vi "ReadSZL.vi"() -> ()   [LabVIEW 2020]
uses:
  lib/Snap7.lvlib
panel:
  out "?":string
  out "SZL List":string
  out "Size":i32
  out "ASCII Data":string
  out "Hex Data":string
  out "Running":bool
  out "Status":string="No Error"
  in  "Index":i32 format="%x"
  in  "ID":i32=17 format="%x"
  in  "?":bool
  in  "Slot":i32=2
  in  "Rack":i32
  in  "Address IP":string="192.168.1.12"
  # "SZL Read"
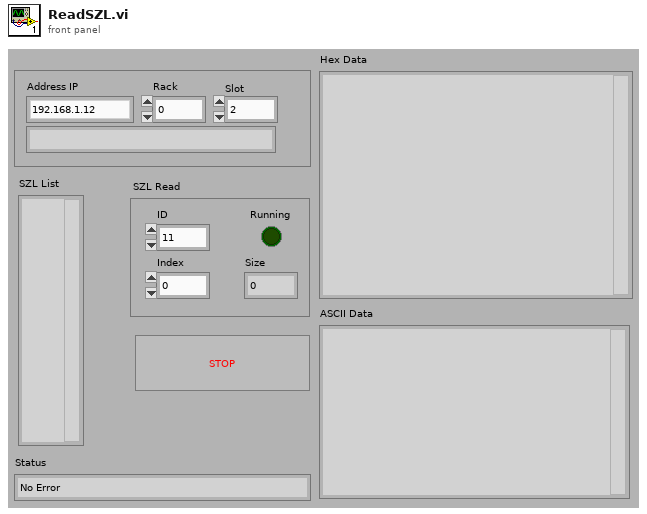
[diagram p1: front panel]
types:
  T1 = enum16{"big-endian, network order", "native, host order", "little-endian"}
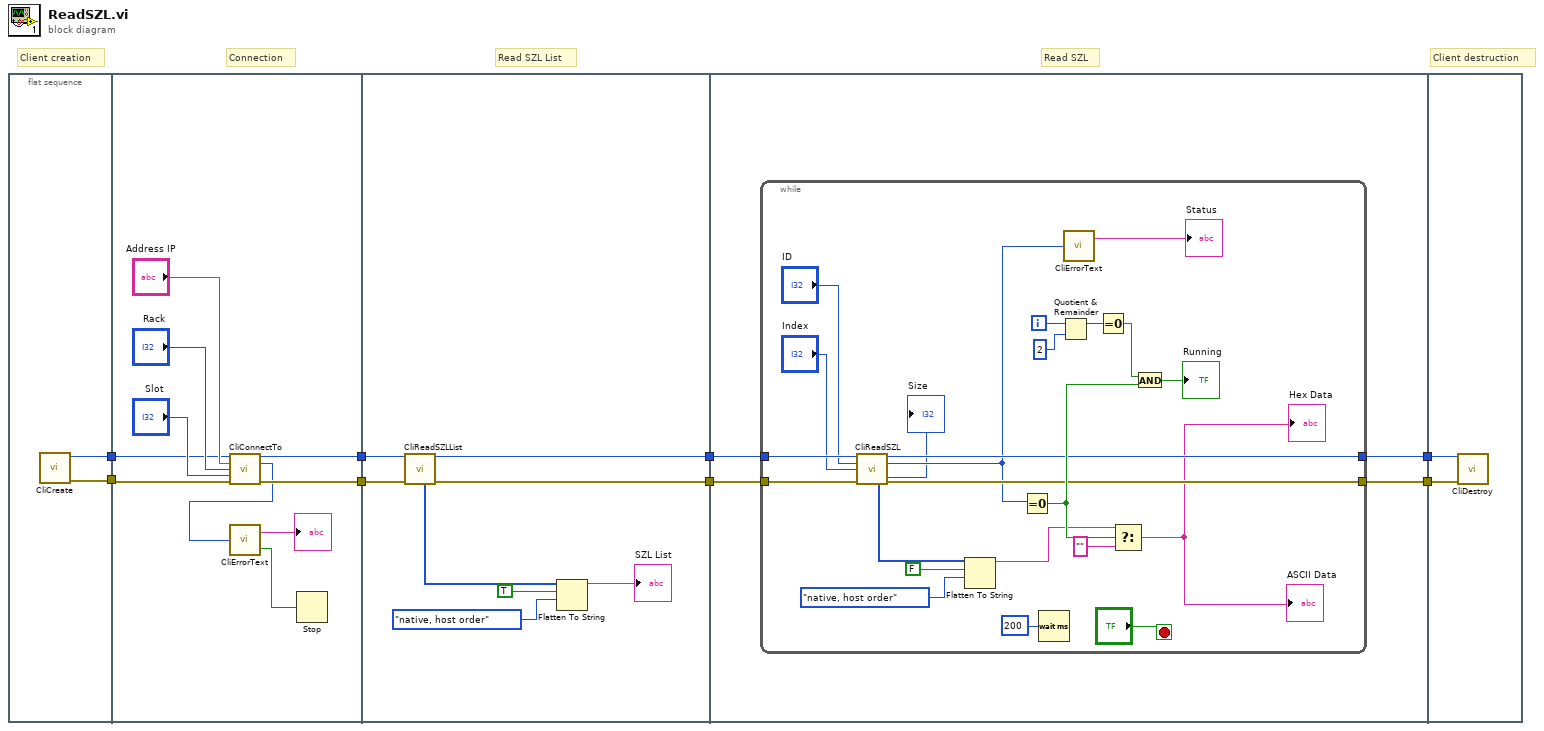
[diagram p0: block diagram]
diagram:
  # "Read SZL List"
  # "Client destruction"
  # "Read SZL"
  # "Connection"
  # "Client creation"
  n1 = flat-sequence {
    tunnel: [w10] -> w8
    tunnel: [w9] -> w7
    tunnel: [w20] -> w4
    tunnel: [w14] -> w2
    tunnel: w8 -> [w16]
    tunnel: w7 -> [w15]
    tunnel: w4 -> [w26]
    tunnel: [w25] -> w3
    tunnel: w2 -> [w28]
    tunnel: [w27] -> w1
    tunnel: w3 -> [w32]
    tunnel: w1 -> [w31]
    tunnel: [w30] -> w6
    tunnel: [w29] -> w5
    tunnel: w6 -> [w57]
    tunnel: w5 -> [w56]
    frame #0 {
      n2 = call "CliCreate.vi"() -> ("ref out"=w10:u64, "error out"=w9:errorcluster)  [unwired: 14 in]
    }
    frame #1 {
      n3 = call "CliConnectTo.vi"("ref in"=w16, "Address"="Address IP", "Rack"="Rack", "Slot"="Slot", "error in (no error)"=w15) -> ("ref out"=w14:u64, "Result"=w12:i32, "error out"=w20:errorcluster)  [unwired: 8 in]
      n4 = call "CliErrorText.vi"("ErrNo"=w12) -> ("Error"=w11:bool, "ErrMessage"=→"?":string)
      n5 = Stop(stop? (T)=w11) -> ()
    }
    frame #2 {
      n6 = call "CliReadSZLList.vi"("ref in"=w28, "error in (no error)"=w26) -> ("ref out"=w27:u64, "List"=w22:u16[], "error out"=w25:errorcluster)  [unwired: 9 in, 2 out]
      n7 = Flatten To String(anything=w22, prepend array or string size? (T)=TRUE, byte order (0:big-endian, network order)=T1."native, host order") -> (data string=→"SZL List":string)  [unwired: 1 in, 2 out]
    }
    frame #3 {
      n8 = while {
        tunnel: w32 -> [w45]
        tunnel: w31 -> [w46]
        tunnel: [w44] -> w30
        tunnel: [w43] -> w29
        i -> [w53]
        stop <- "?" stop-if-true
        n9 = call "CliReadSZL.vi"("ref in"=w46, "ID"="ID", "Index"="Index", "error in (no error)"=w45) -> ("ref out"=w44:u64, "Result"=w42:i32, "Size"=→"Size":i32, "pUsrData"=w38:u8[], "error out"=w43:errorcluster)  [unwired: 5 in, 2 out]
        n10 = Flatten To String(anything=w38, prepend array or string size? (T)=FALSE, byte order (0:big-endian, network order)=T1."native, host order") -> (data string=w40:string)  [unwired: 1 in, 2 out]
        n11 = Equal To 0?(x=w42) -> (x = 0?=w48:bool)
        n12 = Wait (ms)(milliseconds to wait=u32 200 ("Loop Delay (ms)")) -> ()  [unwired: 1 out]
        n13 = Quotient & Remainder(x=w53, y=2) -> (x-y*floor(x/y)=w51:i32)  [unwired: 1 out]
        n14 = call "CliErrorText.vi"("ErrNo"=w42) -> ("ErrMessage"=→"Status":string)  [unwired: 1 out]
        n15 = Equal To 0?(x=w51) -> (x = 0?=w50:bool)
        n16 = Select(t=w40, s=w48, f="") -> (s? t:f=→"ASCII Data" →"Hex Data":string)
        n17 = And(x=w50, y=w48) -> (x .and. y?=→"Running":bool)
      }
    }
    frame #4 {
      n18 = call "CliDestroy.vi"("ref in"=w57, "error in (no error)"=w56) -> ()  [unwired: 13 in, 1 out]
    }
  }
